vi "kdtreesearch.vi"(9 "y":dbl, 10 "x":dbl, 11 "kdtree":dbl[][](array[numeric])) -> (0 "dist":dbl, 1 "yout":dbl, 2 "xout":dbl, 3 "idx":i32, 5 "iter":i32)   [LabVIEW 2012]
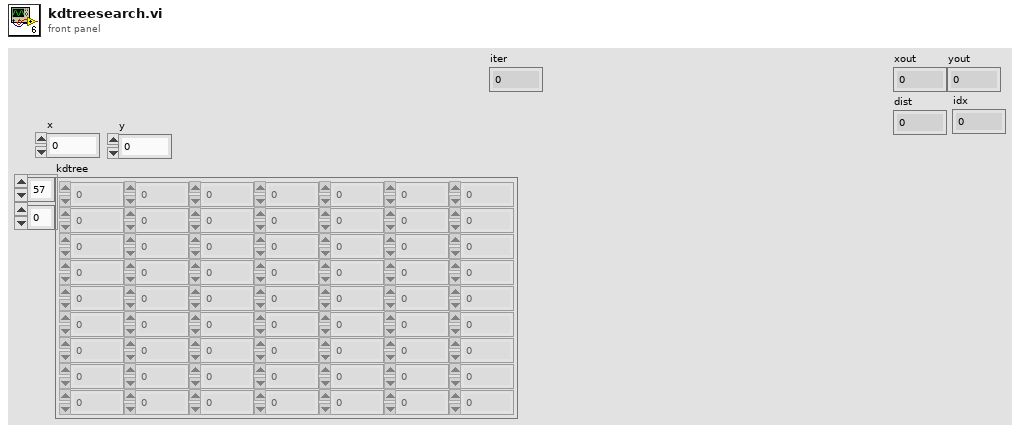
[diagram p1: front panel]
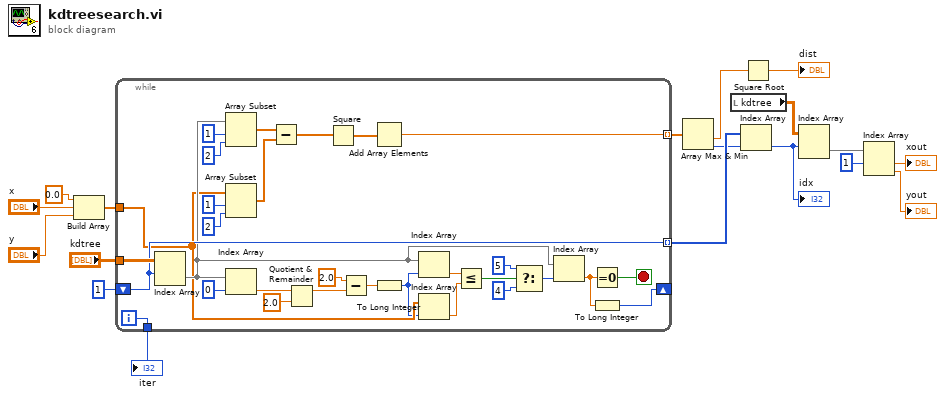
[diagram p0: block diagram]
diagram:
  n1 = Build Array(0.0 ("element"), "x", "y") -> (w13:dbl[])
  n2 = while {
    tunnel: "kdtree" -> [w48]
    shift-right: [w34] -> _
    shift-left: 1 -> [w33]
    tunnel: w13 -> [w27]
    tunnel: [w33] -> w11 mode=indexing
    tunnel: [w22] -> w12 mode=indexing
    tunnel: [w19] -> w1
    i -> [w19]
    stop <- w36 stop-if-true
    n3 = Index Array(array=w48, index (row)=w33) -> (element=w32:dbl[])  [unwired: 1 in]
    n4 = Array Subset(array=w32, index=1, length=2) -> (w26:dbl[])
    n5 = Array Subset(array=w27, index=1, length=2) -> (w25:dbl[])
    n6 = Index Array(array=w32, index=0) -> (element=w46:dbl)
    n7 = Subtract(x=w26, y=w25) -> (x-y=w24:dbl[])
    n8 = Quotient & Remainder(x=w46, y=2.0) -> (x-y*floor(x/y)=w44:dbl)  [unwired: 1 out]
    n9 = Square(x=w24) -> (x^2=w23:dbl[])
    n10 = Subtract(x=2.0 ("y"), y=w44) -> (x-y=w42:dbl)
    n11 = Add Array Elements(numeric array=w23) -> (sum=w22:dbl)
    n12 = To Long Integer(number=w42) -> (32bit integer=w20:i32)
    n13 = Index Array(array=w32, index=w20) -> (element=w41:dbl)
    n14 = Index Array(array=w27, index=w20) -> (element=w21:dbl)
    n15 = Less Or Equal?(x=w41, y=w21) -> (x <= y?=w40:bool)
    n16 = Select(t=5 ("32bit integer"), s=w40, f=4 ("32bit integer")) -> (s? t:f=w37:i32)
    n17 = Index Array(array=w32, index=w37) -> (element=w35:dbl)
    n18 = Equal To 0?(x=w35) -> (x = 0?=w36:bool)
    n19 = To Long Integer(number=w35) -> (32bit integer=w34:i32)
  }
  "iter" <- w1
  n20 = Array Max & Min(array=w12) -> (min value=w5:dbl, min index (indices)=w10:i32)  [unwired: 2 out]
  n21 = local read "kdtree"() -> (w9:dbl[][])
  n22 = Index Array(array=w11, index=w10) -> (element=w8:i32)
  "idx" <- w8
  n23 = Square Root(x=w5) -> (sqrt(x)=→"dist":dbl)
  n24 = Index Array(array=w9, index (row)=w8) -> (element=w7:dbl[])  [unwired: 1 in]
  n25 = Index Array(array=w7, index #1=1 ("index")) -> (element #1=→"xout":dbl, element #2=→"yout":dbl)  [unwired: 1 in]
